vi "MainTester.vi"() -> ()   [LabVIEW 2015]
uses:
  <vilib>/Rock Robotics/WPI/SerialPort/WPI_SerialPortRef.ctl
  <vilib>/Rock Robotics/WPI/SerialPort/WPI_SerialPort.ctl
  Old code/packet types.ctl
panel:
  in  "B 2":dbl(slide) scale=0.0..255.0
  in  "G 2":dbl(slide) scale=0.0..255.0
  in  "R 2":dbl(slide) scale=0.0..255.0
  in  "B":dbl(slide) scale=0.0..255.0
  in  "G":dbl(slide) scale=0.0..255.0
  in  "R":dbl(slide) scale=0.0..255.0
  out "SerialPortRef 6":T1
  out "error out 8":errorcluster
  out "SerialPortRef":T1
  out "error out 7":errorcluster
  in  "Close File 2":bool
  in  "Close File":bool
  in  "Display string":string
  out "error out 6":errorcluster
  out "SerialPortRef 5":T1
  out "ADC voltages":dbl[](array[numeric])
  out "error out 4":errorcluster
  out "SerialPortRef 3":T1
  out "error out 3":errorcluster
  out "SerialPortRef 2":T1
  out "error out 2":errorcluster
  out "All Digital Input Vals":bool[](array[boolean])
  out "error out":errorcluster
  in  "stop":bool
  in  "error in (no error)":errorcluster
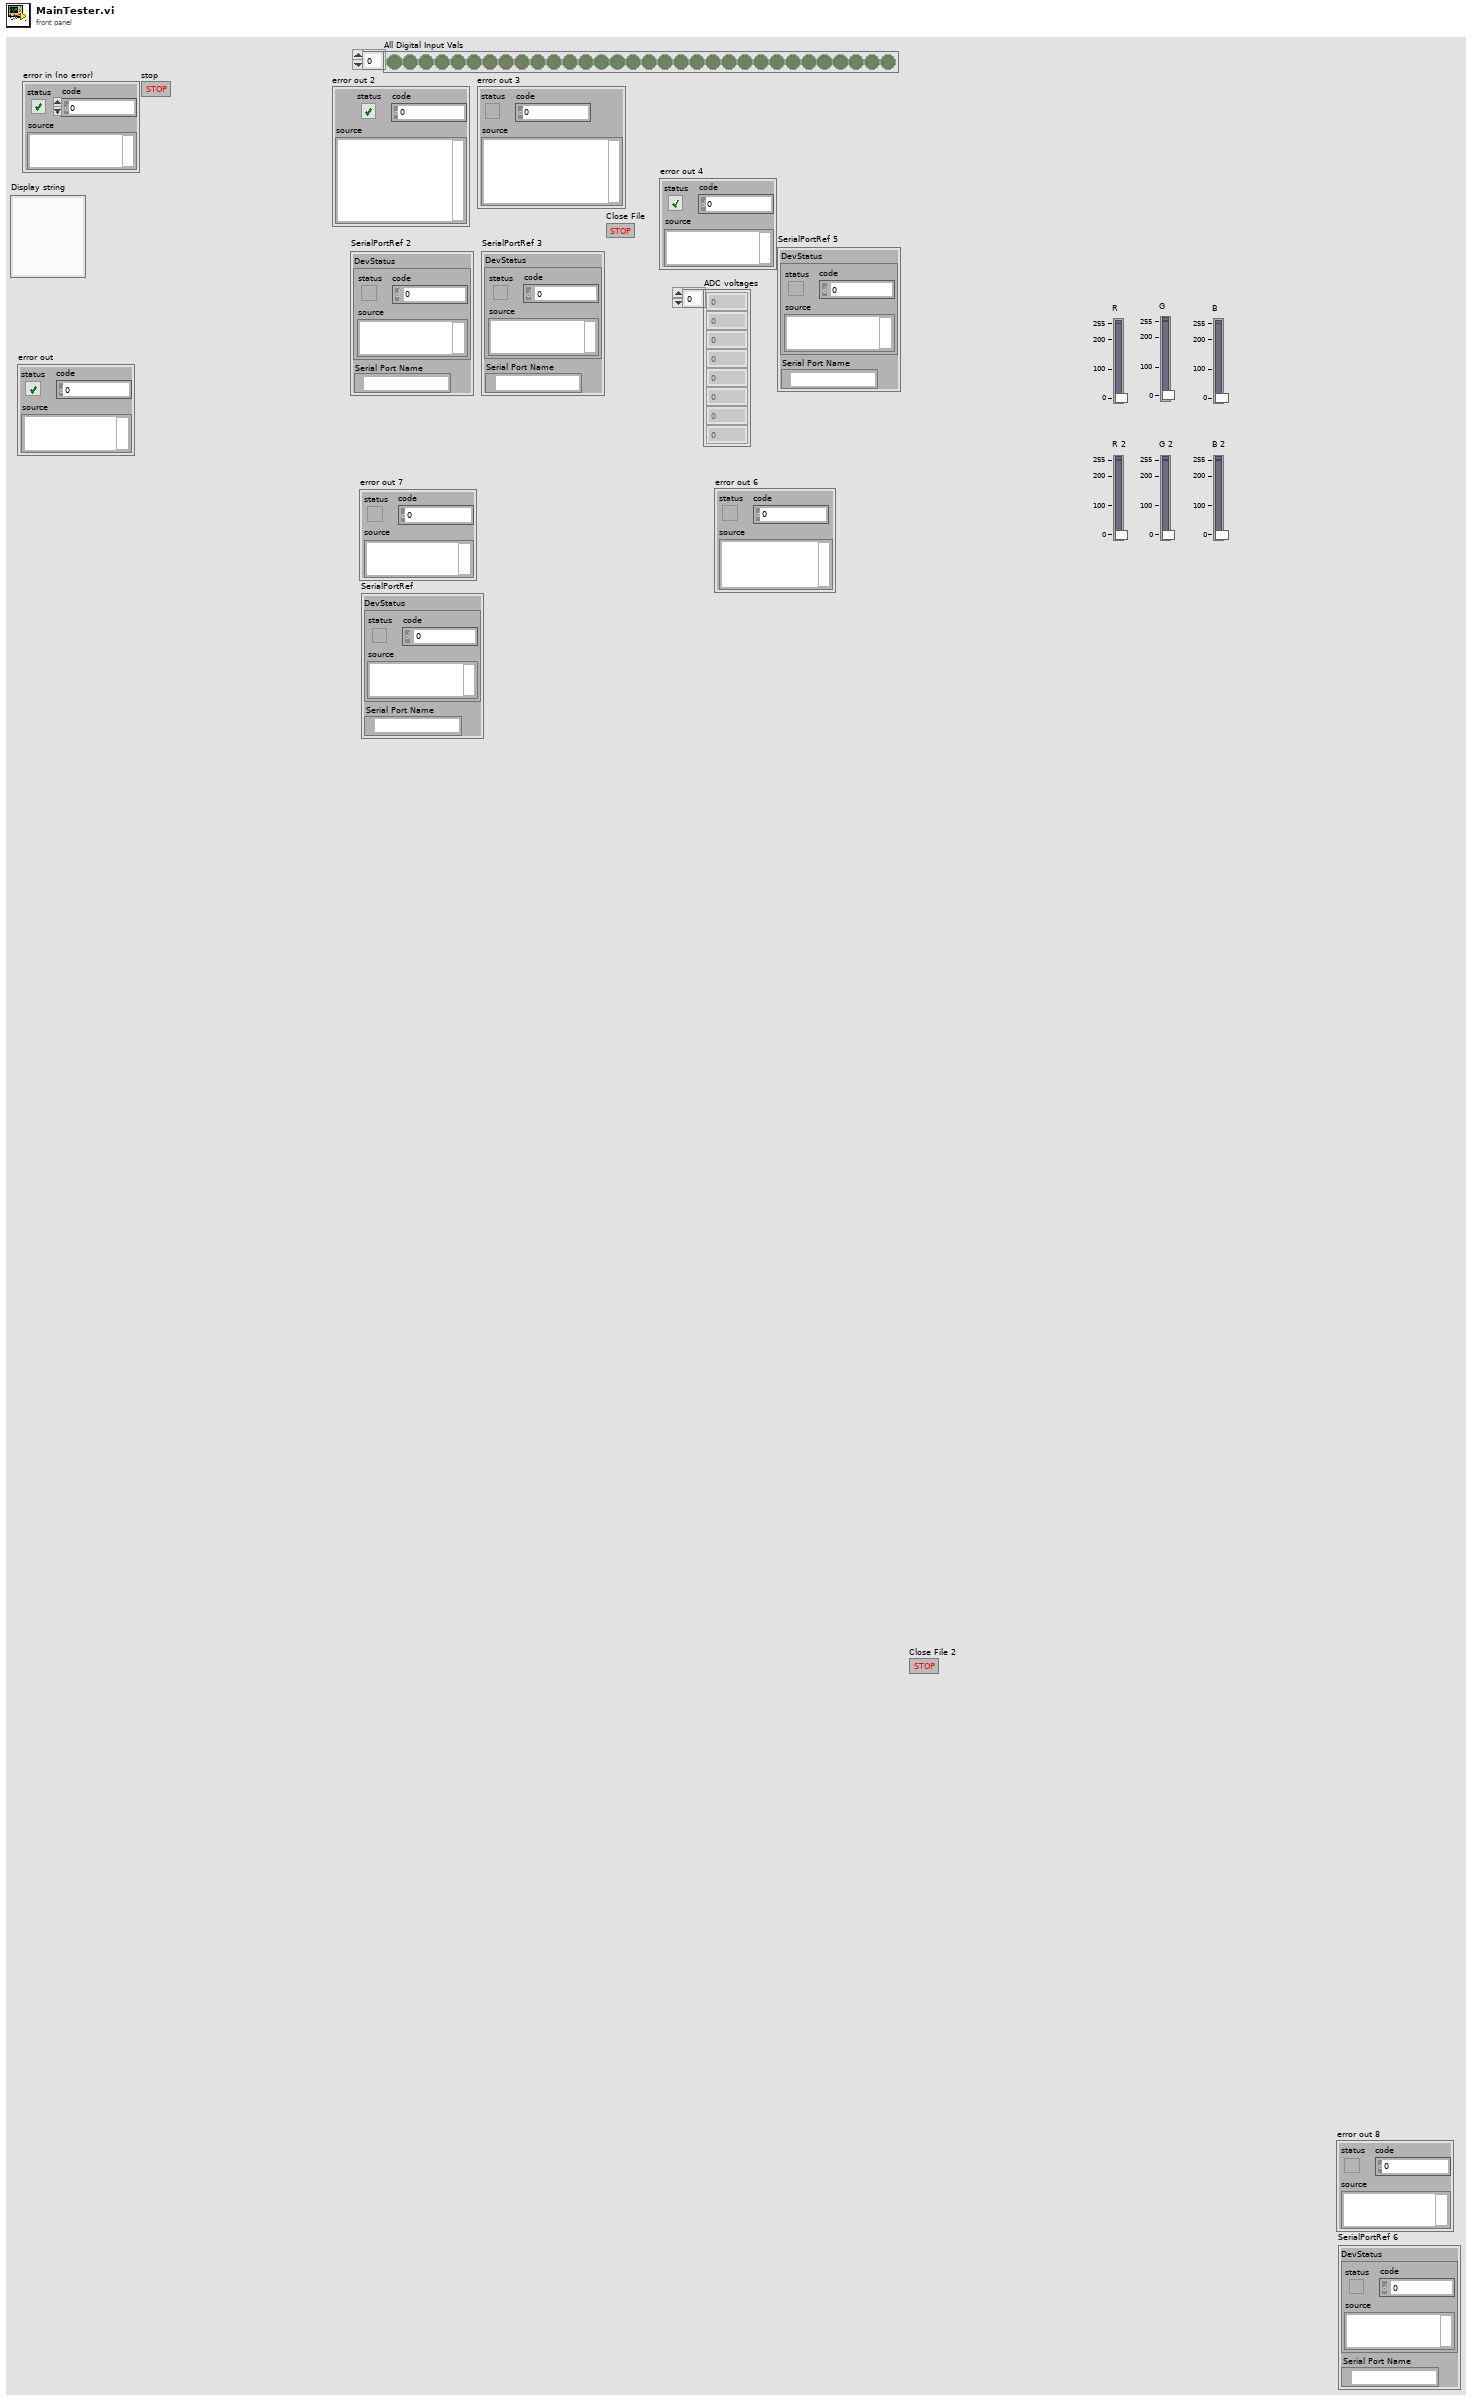
[diagram p1: front panel]
types:
  T1 = typedef "WPI_SerialPortRef.ctl" = cluster{"DevStatus":errorcluster, "Serial Port Name":refnum<visa-resource-name>}
  T2 = typedef "packet types.ctl" = enum16{"Log line", "Open File", "Close File", "Send Header", "Set Time", "Send to LCD"}
  T3 = typedef "WPI_SerialPort.ctl" = enum16{"Onboard RS-232", "MXP TTL"}
  T4 = enum16{"Set Custom RGB", "Set Mode", "Set intensity"}
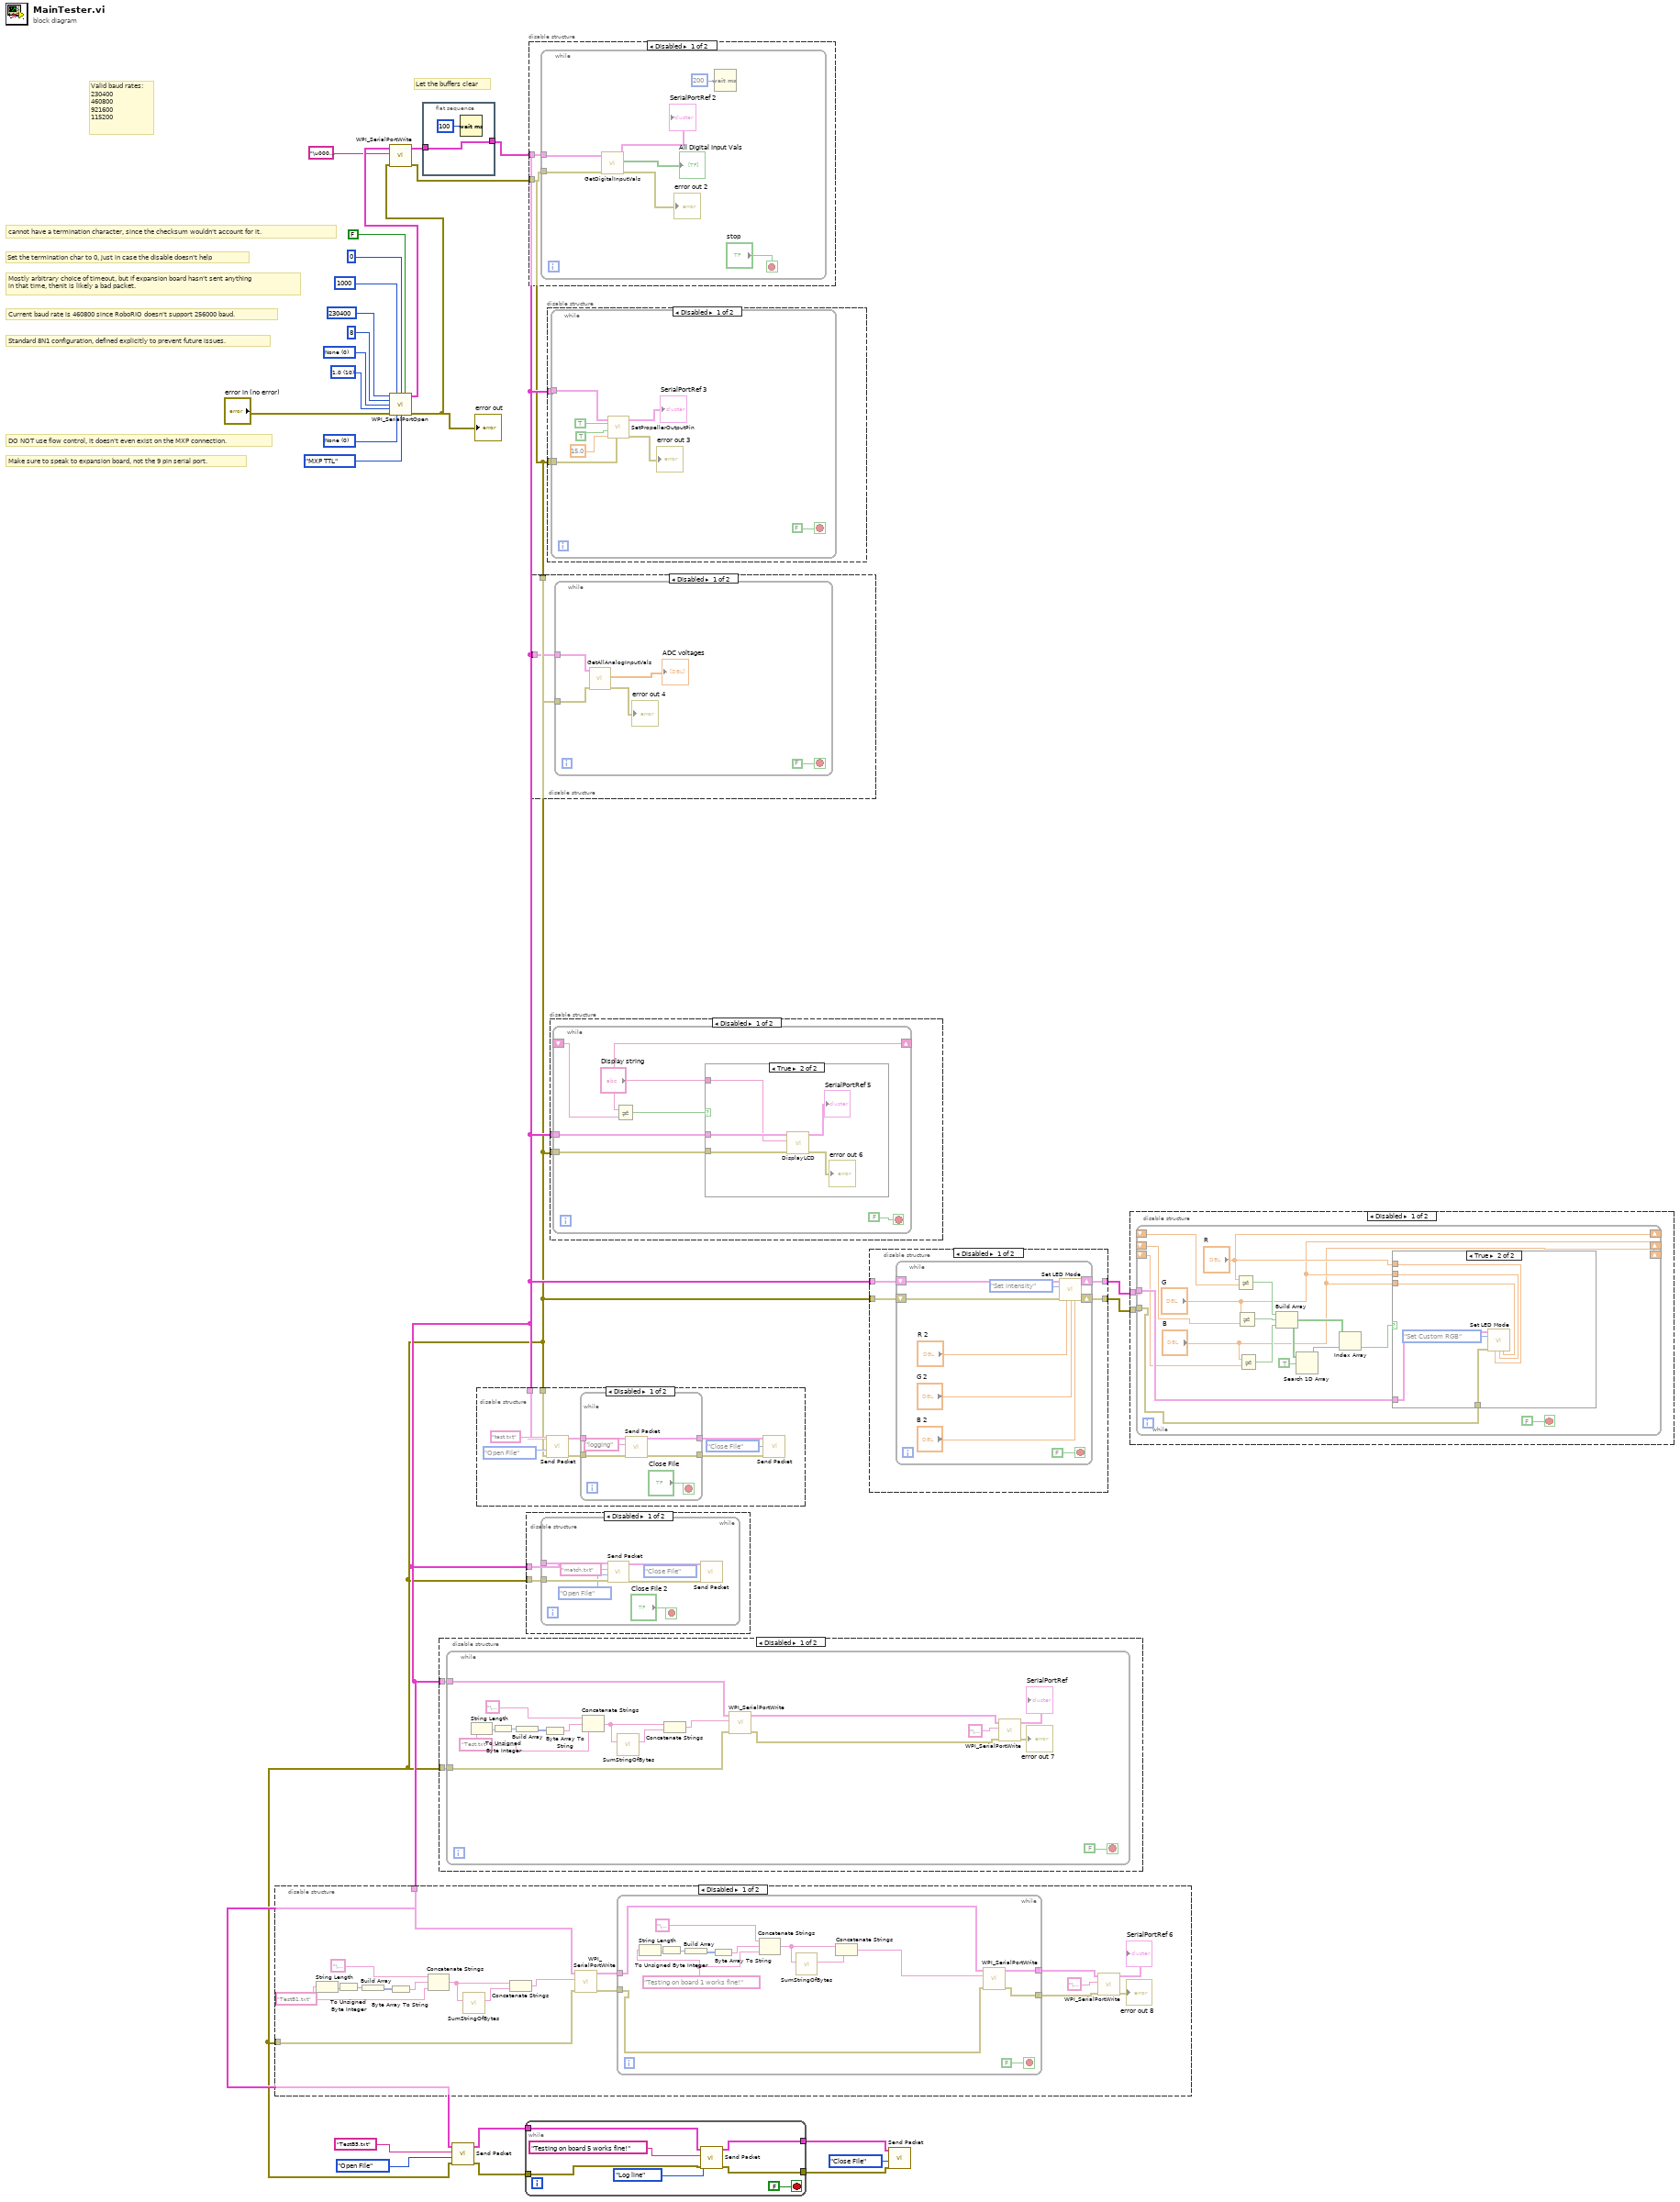
[diagram p0: block diagram]
diagram:
  w24 = u16 10 items=["1.0"=10, "1.5"=15, "2.0"=20] ("Stop Bits")
  w20 = u16 0 items=["None", "XON/XOFF", "RTS/CTS", "XON/XOFF & RTS/CTS", "DTR/DSR", "XON/XOFF & DTR/DSR"] ("Flow Control")
  w19 = u16 0 items=["None", "Odd", "Even", "Mark", "Space"] ("Parity")
  # "Let the buffers clear"
  # "Valid baud rates:\n230400\n460800\n921600\n115200"
  # "Make sure to speak to expansion board, not the 9 pin serial port."
  # "DO NOT use flow control, it doesn't even exist on the MXP connection."
  # "Standard 8N1 configuration, defined explicitly to prevent future issues."
  # "Current baud rate is 460800 since RoboRIO doesn't support 256000 baud."
  # "Mostly arbitrary choice of timeout, but if expansion board hasn't sent anything\nin that time, thenit is likely a bad packet."
  # "Set the termination char to 0, just in case the disable doesn't help"
  # "cannot have a termination character, since the checksum wouldn't account for it."
  n1 = call <vilib>:"WPI_SerialPortOpen.vi"("Baud Rate"=u32 230400, "Timeout Value (ms)"=u32 1000, "Termination Char (0xA = '\\n' = LF)"=u8 0 ("Termination Char (0xA = '\\n' = LF)"), "Enable Termination Char? (T)"=FALSE, "Data Bits"=u16 8, "Parity"=w19, "Stop Bits"=w24, "error in (no error)"="error in (no error)", "Flow Control"=w20, "Serial Port"=WPI_SerialPort."MXP TTL") -> ("SerialPortRef"=w15:T1, "error out"=w14:errorcluster)  [unwired: 4 in]
  "error out" <- w14
  n2 = call <vilib>:"WPI_SerialPortWrite.vi"("error in (no error)"=w14, "Buffer"="\u0004\u0004", "SerialPortRef"=w15) -> ("error out"=w8:errorcluster, "SerialPortRef"=w12:T1)  [unwired: 6 in, 1 out]
  n3 = disable-structure shown="Disabled" {
    disable-tunnel: w9 -> [w27 _]
    disable-tunnel: w8 -> [w26 _]
    frame Disabled {
      w28 = "TestB1.txt"
      n4 = String Length(string=w28) -> (length=w36:i32)
      n5 = To Unsigned Byte Integer(number=w36) -> (unsigned 8bit integer=w39:u8)
      n6 = Build Array(w39) -> (w38:u8[])
      n7 = Byte Array To String(unsigned byte array=w38) -> (string=w37:string)
      n8 = Concatenate Strings("\u0003", w37, w28) -> (w42:string)
      n9 = call "SumStringOfBytes.vi"("String Of Bytes"=w42) -> ("SumAsString"=w43:string)  [unwired: 10 in]
      n10 = Concatenate Strings(w42, w43) -> (w40:string)
      n11 = call <vilib>:"WPI_SerialPortWrite.vi"("error in (no error)"=w26, "Buffer"=w40, "SerialPortRef"=w27) -> ("error out"=w34:errorcluster, "SerialPortRef"=w35:T1)  [unwired: 6 in, 1 out]
      n12 = while {
        tunnel: w35 -> [w57]
        tunnel: w34 -> [w56]
        tunnel: [w46] -> w30
        tunnel: [w45] -> w29
        stop <- FALSE stop-if-true
        w50 = "Testing on board 1 works fine!"
        n13 = String Length(string=w50) -> (length=w52:i32)
        n14 = To Unsigned Byte Integer(number=w52) -> (unsigned 8bit integer=w54:u8)
        n15 = Build Array(w54) -> (w53:u8[])
        n16 = Byte Array To String(unsigned byte array=w53) -> (string=w51:string)
        n17 = Concatenate Strings("\u0001", w51, w50) -> (w48:string)
        n18 = call "SumStringOfBytes.vi"("String Of Bytes"=w48) -> ("SumAsString"=w49:string)  [unwired: 10 in]
        n19 = Concatenate Strings(w48, w49) -> (w47:string)
        n20 = call <vilib>:"WPI_SerialPortWrite.vi"("error in (no error)"=w56, "Buffer"=w47, "SerialPortRef"=w57) -> ("error out"=w45:errorcluster, "SerialPortRef"=w46:T1)  [unwired: 6 in, 1 out]
      }
      n21 = call <vilib>:"WPI_SerialPortWrite.vi"("error in (no error)"=w29, "Buffer"="\u0004", "SerialPortRef"=w30) -> ("error out"=→"error out 8":errorcluster, "SerialPortRef"=→"SerialPortRef 6":T1)  [unwired: 6 in, 1 out]
    }
    frame Enabled {
    }
  }
  n22 = flat-sequence {
    tunnel: [w59] -> w9
    tunnel: w12 -> [w59]
    frame #0 {
      n23 = Wait (ms)(milliseconds to wait=u32 100) -> ()  [unwired: 1 out]
    }
  }
  n24 = disable-structure shown="Disabled" {
    disable-tunnel: w8 -> [w61 _]
    disable-tunnel: w9 -> [w60 _]
    frame Disabled {
      n25 = while {
        tunnel: w60 -> [w78]
        tunnel: w61 -> [w77]
        stop <- FALSE stop-if-true
        w68 = "Test.txt"
        n26 = String Length(string=w68) -> (length=w64:i32)
        n27 = To Unsigned Byte Integer(number=w64) -> (unsigned 8bit integer=w67:u8)
        n28 = Build Array(w67) -> (w66:u8[])
        n29 = Byte Array To String(unsigned byte array=w66) -> (string=w65:string)
        n30 = Concatenate Strings("\u0003", w65, w68) -> (w75:string)
        n31 = call "SumStringOfBytes.vi"("String Of Bytes"=w75) -> ("SumAsString"=w76:string)  [unwired: 10 in]
        n32 = Concatenate Strings(w75, w76) -> (w73:string)
        n33 = call <vilib>:"WPI_SerialPortWrite.vi"("error in (no error)"=w77, "Buffer"=w73, "SerialPortRef"=w78) -> ("error out"=w62:errorcluster, "SerialPortRef"=w63:T1)  [unwired: 6 in, 1 out]
        n34 = call <vilib>:"WPI_SerialPortWrite.vi"("error in (no error)"=w62, "Buffer"="\u0004", "SerialPortRef"=w63) -> ("error out"=→"error out 7":errorcluster, "SerialPortRef"=→"SerialPortRef":T1)  [unwired: 6 in, 1 out]
      }
    }
    frame Enabled {
    }
  }
  n35 = call "Send Packet.vi"("error in (no error) 2"=w8, 7:packet_types."Open File", "Log string 2"="TestB5.txt", "SerialPortRef 2"=w9) -> ("error out 2"=w4:errorcluster, "SerialPortRef out 2"=w5:T1)  [unwired: 4 in]
  n36 = disable-structure shown="Disabled" {
    disable-tunnel: w9 -> [w80 _]
    disable-tunnel: w8 -> [w79 _]
    frame Disabled {
      n37 = call "Send Packet.vi"("error in (no error) 2"=w79, 7:packet_types."Open File", "Log string 2"="test.txt" ("Log string"), "SerialPortRef 2"=w80) -> ("error out 2"=w84:errorcluster, "SerialPortRef out 2"=w85:T1)  [unwired: 4 in]
      n38 = while {
        tunnel: w85 -> [w93]
        tunnel: w84 -> [w92]
        tunnel: [w89] -> w83
        tunnel: [w88] -> w82
        stop <- "Close File" stop-if-true
        n39 = call "Send Packet.vi"("error in (no error) 2"=w92, "Log string 2"="logging" ("Log string"), "SerialPortRef 2"=w93) -> ("error out 2"=w88:errorcluster, "SerialPortRef out 2"=w89:T1)  [unwired: 5 in]
      }
      n40 = call "Send Packet.vi"("error in (no error) 2"=w82, 7:packet_types."Close File", "SerialPortRef 2"=w83) -> ()  [unwired: 5 in, 2 out]
    }
    frame Enabled {
    }
  }
  n41 = while {
    tunnel: w5 -> [w97]
    tunnel: w4 -> [w94]
    tunnel: [w96] -> w2
    tunnel: [w95] -> w1
    stop <- FALSE stop-if-true
    n42 = call "Send Packet.vi"("error in (no error) 2"=w94, 7:packet_types."Log line", "Log string 2"="Testing on board 5 works fine!", "SerialPortRef 2"=w97) -> ("error out 2"=w95:errorcluster, "SerialPortRef out 2"=w96:T1)  [unwired: 4 in]
  }
  n43 = disable-structure shown="Disabled" {
    disable-tunnel: w9 -> [w102 _]
    disable-tunnel: w8 -> [w101 _]
    frame Disabled {
      n44 = while {
        tunnel: w102 -> [w109]
        tunnel: w101 -> [w108]
        stop <- "Close File 2" stop-if-true
        (unwired) packet_types."Close File"
        n45 = call "Send Packet.vi"("error in (no error) 2"=w108, 7:packet_types."Open File", "Log string 2"="match.txt" ("Log string"), "SerialPortRef 2"=w109) -> ("error out 2"=w103:errorcluster, "SerialPortRef out 2"=w104:T1)  [unwired: 4 in]
        n46 = call "Send Packet.vi"("error in (no error) 2"=w103, "SerialPortRef 2"=w104) -> ()  [unwired: 6 in, 2 out]
      }
    }
    frame Enabled {
    }
  }
  n47 = disable-structure shown="Disabled" {
    disable-tunnel: w9 -> [w111 _]
    disable-tunnel: w8 -> [w110 _]
    frame Disabled {
      n48 = while {
        tunnel: w110 -> [w116]
        tunnel: w111 -> [w117]
        stop <- "stop" stop-if-true
        n49 = call "GetDigitalInputVals.vi"("error in (no error)"=w116, "SerialPortRef"=w117) -> ("error out"=→"error out 2":errorcluster, "All Digital Input Vals"=→"All Digital Input Vals":bool[], "SerialPortRef 2"=→"SerialPortRef 2":T1)  [unwired: 7 in]
        n50 = Wait (ms)(milliseconds to wait=u32 200) -> ()  [unwired: 1 out]
      }
    }
    frame Enabled {
    }
  }
  n51 = disable-structure shown="Disabled" {
    disable-tunnel: w9 -> [w120 _]
    disable-tunnel: w8 -> [w119 _]
    frame Disabled {
      n52 = while {
        tunnel: w120 -> [w125]
        tunnel: w119 -> [w124]
        stop <- FALSE stop-if-true
        n53 = call "GetAllAnalogInputVals.vi"("error in (no error)"=w124, "SerialPortRef"=w125) -> ("error out"=→"error out 4":errorcluster, "ADC voltages"=→"ADC voltages":dbl[])  [unwired: 6 in, 2 out]
      }
    }
    frame Enabled {
    }
  }
  n54 = disable-structure shown="Disabled" {
    disable-tunnel: w9 -> [w127 _]
    disable-tunnel: w8 -> [w126 _]
    frame Disabled {
      n55 = while {
        tunnel: w126 -> [w132]
        tunnel: w127 -> [w129]
        stop <- FALSE stop-if-true
        n56 = call "SetPropellerOutputPin.vi"("error in (no error)"=w132, "Pin Number"=15.0, "Value"=TRUE, "Dir"=TRUE, "SerialPortRef"=w129) -> ("error out"=→"error out 3":errorcluster, "SerialPortRef 2"=→"SerialPortRef 3":T1)  [unwired: 5 in]
      }
    }
    frame Enabled {
    }
  }
  n57 = disable-structure shown="Disabled" {
    disable-tunnel: w9 -> [w137 _]
    disable-tunnel: w8 -> [w136 _]
    frame Disabled {
      n58 = while {
        tunnel: w137 -> [w141]
        tunnel: w136 -> [w143]
        shift-right: ["Display string"] -> _
        shift-left: _ -> [w139]
        stop <- FALSE stop-if-true
        n59 = Not Equal?(x="Display string", y=w139) -> (x != y?=w138:bool)
        n60 = case shown="True" w138 {
          tunnel: w141 -> [_ w148]
          tunnel: w143 -> [_ w147]
          tunnel: "Display string" -> [_ w144]
          frame False {
          }
          frame True {
            n61 = call "DisplayLCD.vi"("error in (no error)"=w147, "Display string"=w144, "SerialPortRef"=w148) -> ("error out"=→"error out 6":errorcluster, "SerialPortRef 2"=→"SerialPortRef 5":T1)  [unwired: 7 in]
          }
        }
      }
    }
    frame Enabled {
    }
  }
  n62 = disable-structure shown="Disabled" {
    disable-tunnel: w8 -> [w152 _]
    disable-tunnel: w9 -> [w151 _]
    disable-tunnel: [w150 _] -> w11
    disable-tunnel: [w149 _] -> w10
    frame Disabled {
      n63 = while {
        shift-right: [w158] -> w149
        shift-left: w152 -> [w161]
        shift-right: [w159] -> w150
        shift-left: w151 -> [w160]
        stop <- FALSE stop-if-true
        n64 = call "Set LED Mode.vi"("SerialPortRef 3"=w160, 5:T4."Set intensity" ("Enum"), "error in (no error)"=w161, "Red"="R 2", "Green"="G 2", "Blue"="B 2") -> ("SerialPortRef"=w159:T1, "error out"=w158:errorcluster)  [unwired: 8 in]
      }
    }
    frame Enabled {
    }
  }
  n65 = call "Send Packet.vi"("error in (no error) 2"=w1, 7:packet_types."Close File", "SerialPortRef 2"=w2) -> ()  [unwired: 5 in, 2 out]
  n66 = disable-structure shown="Disabled" {
    disable-tunnel: w11 -> [w163 _]
    disable-tunnel: w10 -> [w162 _]
    frame Disabled {
      n67 = while {
        tunnel: w163 -> [w177]
        tunnel: w162 -> [w178]
        shift-right: ["R"] -> _
        shift-left: _ -> [w176]
        shift-right: ["G"] -> _
        shift-left: _ -> [w175]
        shift-right: ["B"] -> _
        shift-left: _ -> [w174]
        stop <- FALSE stop-if-true
        n68 = Not Equal?(x="R", y=w176) -> (x != y?=w171:bool)
        n69 = Not Equal?(x="G", y=w175) -> (x != y?=w173:bool)
        n70 = Not Equal?(x="B", y=w174) -> (x != y?=w172:bool)
        n71 = Build Array(w171, w173, w172) -> (w168:bool[])
        n72 = Search 1D Array(1D array=w168, element=TRUE) -> (index of element=w169:i32)  [unwired: 1 in]
        n73 = Index Array(array=w168, index=w169) -> (element=w167:bool)
        n74 = case shown="True" w167 {
          tunnel: w178 -> [_ w184]
          tunnel: w177 -> [_ w185]
          tunnel: "R" -> [_ w180]
          tunnel: "G" -> [_ w181]
          tunnel: "B" -> [_ w182]
          frame False {
          }
          frame True {
            n75 = call "Set LED Mode.vi"("SerialPortRef 3"=w185, 5:enum16{"Set Custom RGB", "Set Mode"}."Set Custom RGB" ("Enum"), "error in (no error)"=w184, "Red"=w180, "Green"=w181, "Blue"=w182) -> ()  [unwired: 8 in, 2 out]
          }
        }
      }
    }
    frame Enabled {
    }
  }
